vi "taskqueue ref.vi"(8 "错误输入（无错误）":errorcluster) -> (0 "错误输出":errorcluster, 3 "队列输出":refnum<queue>)   [LabVIEW 2022 SP3, in "斯坦道CODcr.lvlib"]
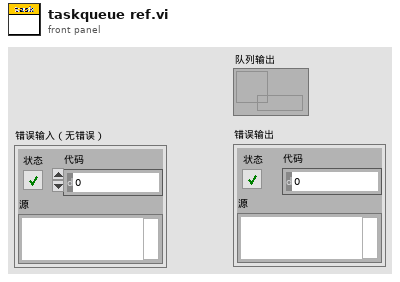
[diagram p1: front panel]
types:
  T1 = typedef "控制命令与参数.ctl" = cluster{"控制命令":enum16{"启动测量", "标样核查", "零点核查", "跨度核查", "空白测试", "平行样测试", "加标回收", "空白校准", "标样校准", "初始化（清洗）", "停止测试", "仪器重启", "校时", "模式设置", "测量间隔设置"}, "测量参数":string}
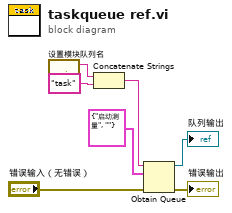
[diagram p0: block diagram]
diagram:
  n1 = call "设置模块队列名.vi"() -> ("Msg"=w7:string)  [unwired: 5 in]
  n2 = Concatenate Strings(w7, "task" ("字符串")) -> (w5:string)
  n3 = Obtain Queue(name (unnamed)=w5, element data type=T1 {"控制命令"=enum."启动测量", "测量参数"=""} ("输入参数"), error in (no error)="错误输入（无错误）") -> (queue out=→"队列输出":refnum<queue>, error out=→"错误输出":errorcluster)  [unwired: 2 in, 1 out]
